vi "DataTranslation.vi"() -> ()   [LabVIEW 2014]
doc: "This vi will take data with multiple DT boxes for an arbitrary number of channels either differentially or single ended, depending upon how you have wired the boxes up."
uses:
  Controls/DT_Cluster.ctl
  Controls/DT_Mode.ctl
  Globals/Meas_global.vi
  Globals/Dynamic_call_global.ph.vi
  Globals/Trav_pos_global.vi
  Globals/Extra_Commands_Global.vi
  <userlib>/LV-Link3/PolySubVIs/DtCreateAinChan.vi
  <userlib>/LV-Link3/PolySubVIs/DtCreateCtrRateChan.vi
  <userlib>/LV-Link3/PolySubVIs/DtOLTimingSetInput.vi
  <userlib>/LV-Link3/PolySubVIs/DtOLStartNormal.vi
  <userlib>/LV-Link3/PolySubVIs/DtOLTriggerDigital.vi
  <userlib>/LV-Link3/PolySubVIs/DtOLReadMultiple2D.vi
panel:
  out "DAQ Error":errorcluster
  out "Array":T1[](array[typedef])
  out "Waveform Graph":dbl[][](graph)
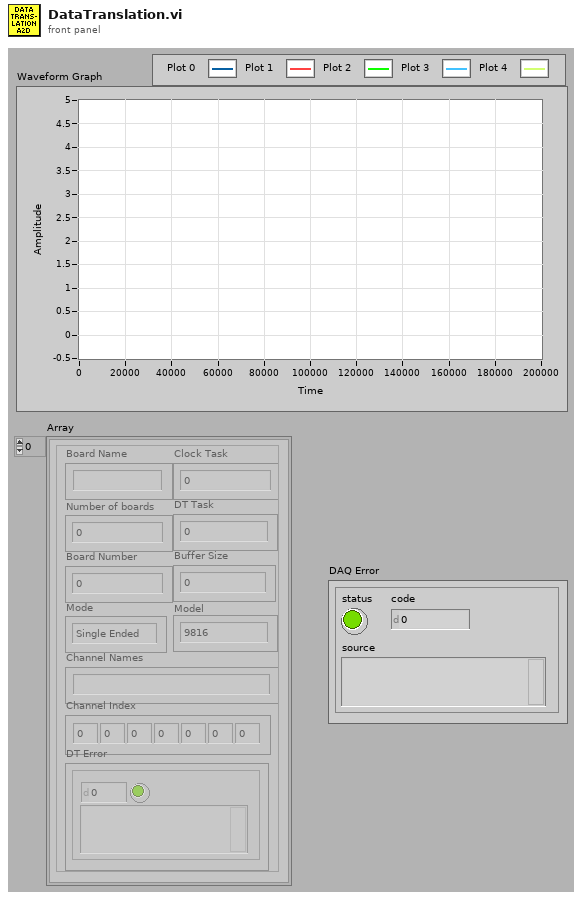
[diagram p1: front panel]
types:
  T1 = typedef "DT_Cluster.ctl" = cluster{"Board Name":string, "Number of boards":u32, "Board Number":u32, "Channel Names":string, "Channel Index":i32[], "DT Task":i32, "DT Error":errorcluster, "Mode":T2, "Buffer Size":u32, "Clock Task":i32, "Model":enum16{"9816", "9836", "9853"}}
  T2 = typedef "DT_Mode.ctl" = enum16{"Single Ended", "Differential"}
  T3 = typedef "Trigger_Mode.ctl" = enum16{"Free Running", "Start on Trigger", "Trigger Every Block", "Trigger Every Sample"}
  T4 = typedef "LDA_Setup.ctl" = cluster{"dimensions":enum16{"1D", "2D"}, "Analogue Freq Multiplier":dbl}
  T5 = enum32{"Internal Clock", "External Clock", "No Timing"}
  T6 = typedef "Traverse_cluster.ctl" = cluster{"Start X":dbl, "Start Y":dbl, "Start Z":dbl, "End X":dbl, "End Y":dbl, "End Z":dbl, "No. of pts.":i32, "Spacing":T7, "Filename":path, "Tunnel Speed":dbl, "Averaging time (min)":dbl, "Extra Commands":string, "Specific Arguments":string, "Emission Rate (l/min)":dbl, "Trace Gas Concentration (%)":dbl, "Density Ratio":string, "Comments":string, "Row No":i32, "Row Type Selector":T8, "Completion time":string, "Row Duration (mins)":dbl, "No. of Valid pts.":i32, "Meas Setup File":string}
  T7 = typedef "Spacing.ctl" = enum16{"Linear", "Log", "Gauss", "Specified", "N/A"}
  T8 = typedef "Multi_run_mode.ctl" = enum16{"Move Traverse Only", "Set Tunnel Speed Only", "Set Source Only", "Set Measurement Conditions", "Single Measurement", "Vertical Profile", "Lateral Profile", "Longitudinal Profile", "Explore Volume", "Multi-Axis Profile", "Auto Calibrate", "Meas Fast FID Bkgnd", "Check Beam Power", "Scanning Valve Measurement", "Run VI Named:", "Set ADAM Ch", "Wait (minutes)", "Send Message", "Synchronize With:", "Fall Back to this Row", "Turn Off Row Repeating", "Blank Row", "Traverse 3D Volume"}
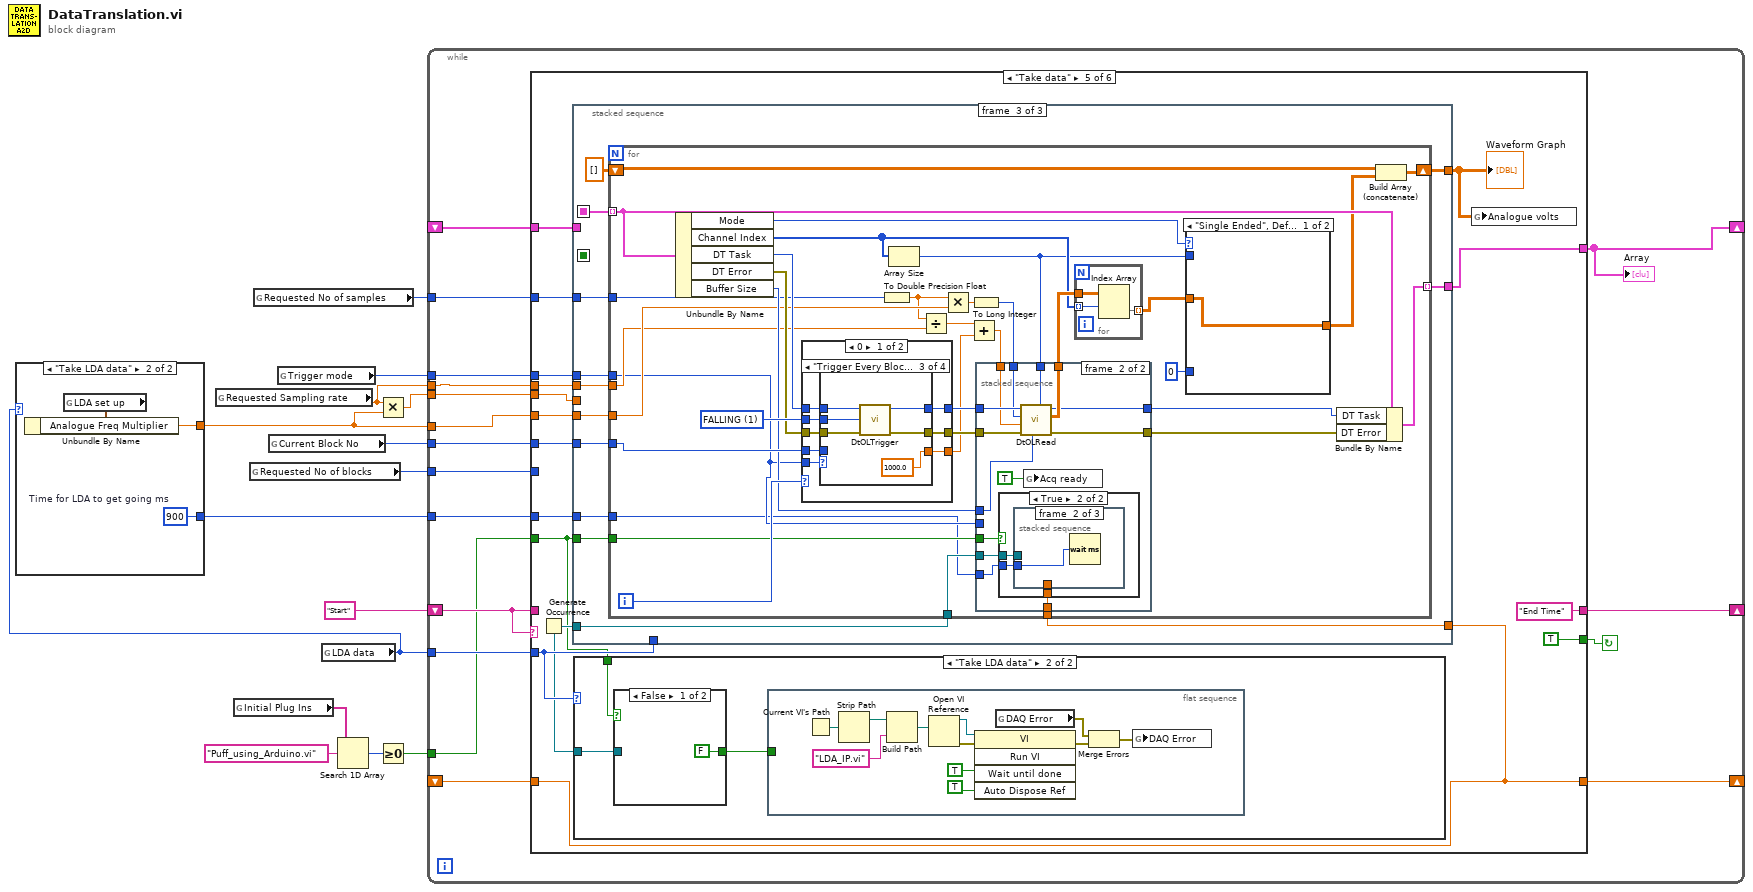
[diagram p0: block diagram]
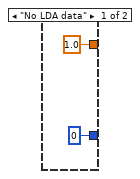
[diagram p2: hidden frame]
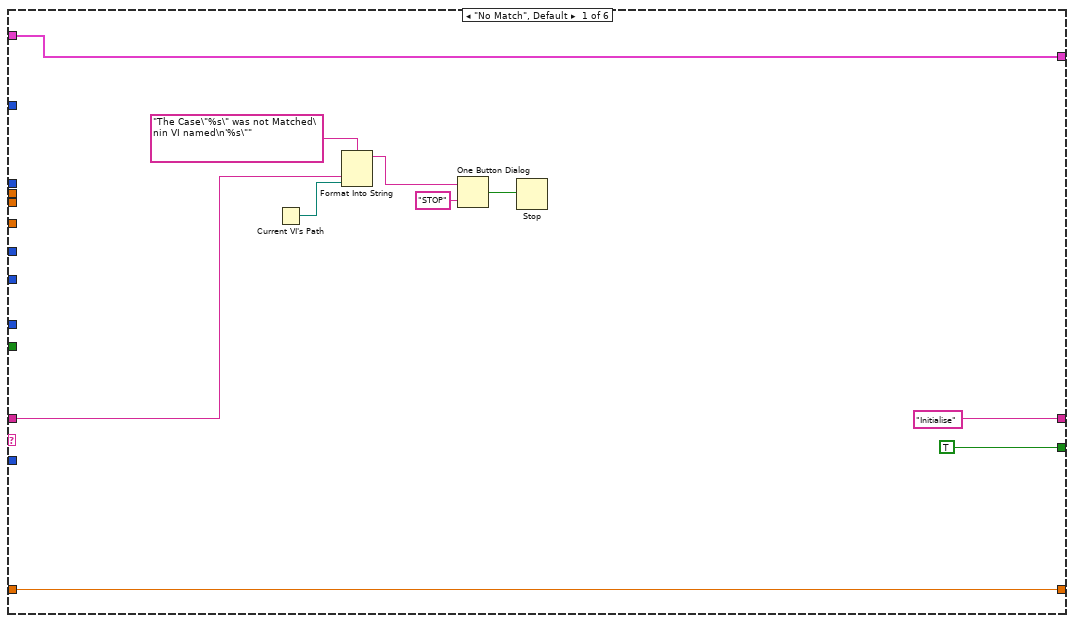
[diagram p3: hidden frame]
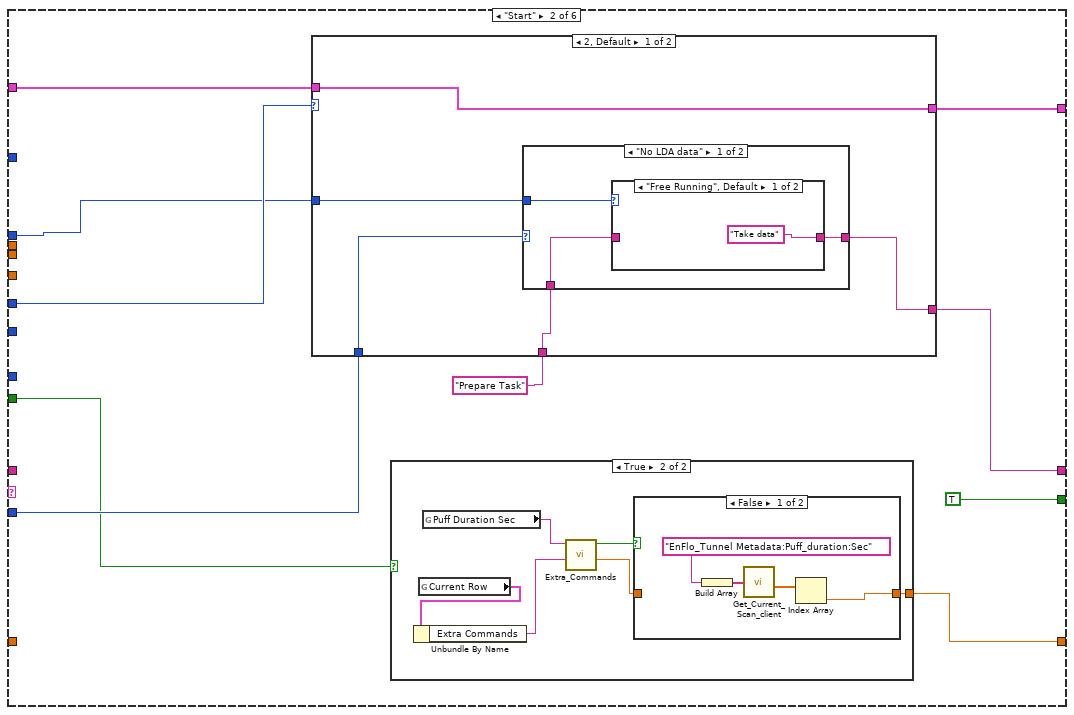
[diagram p4: hidden frame]
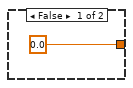
[diagram p5: hidden frame]
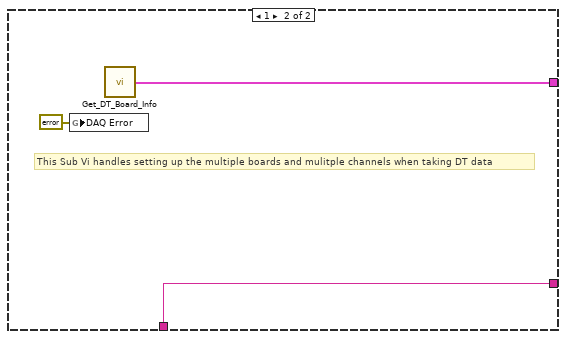
[diagram p9: hidden frame]
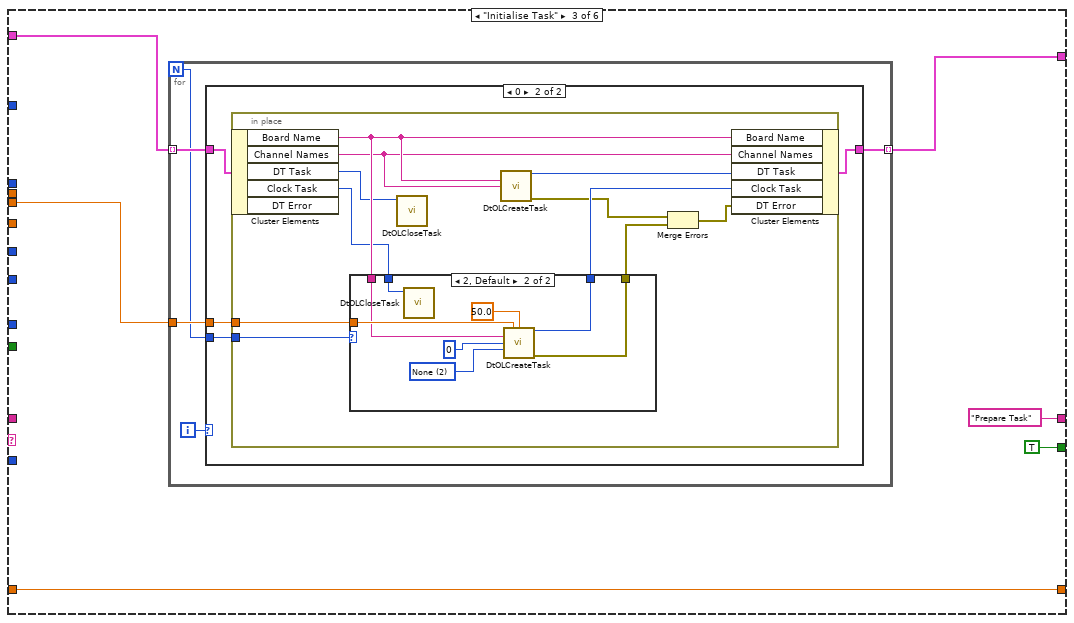
[diagram p10: hidden frame]
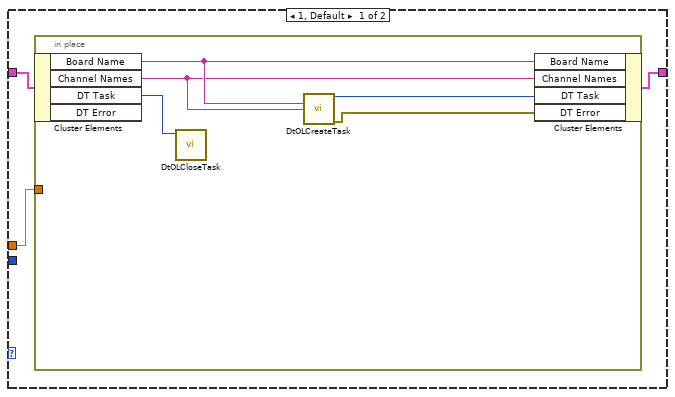
[diagram p11: hidden frame]
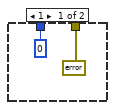
[diagram p12: hidden frame]
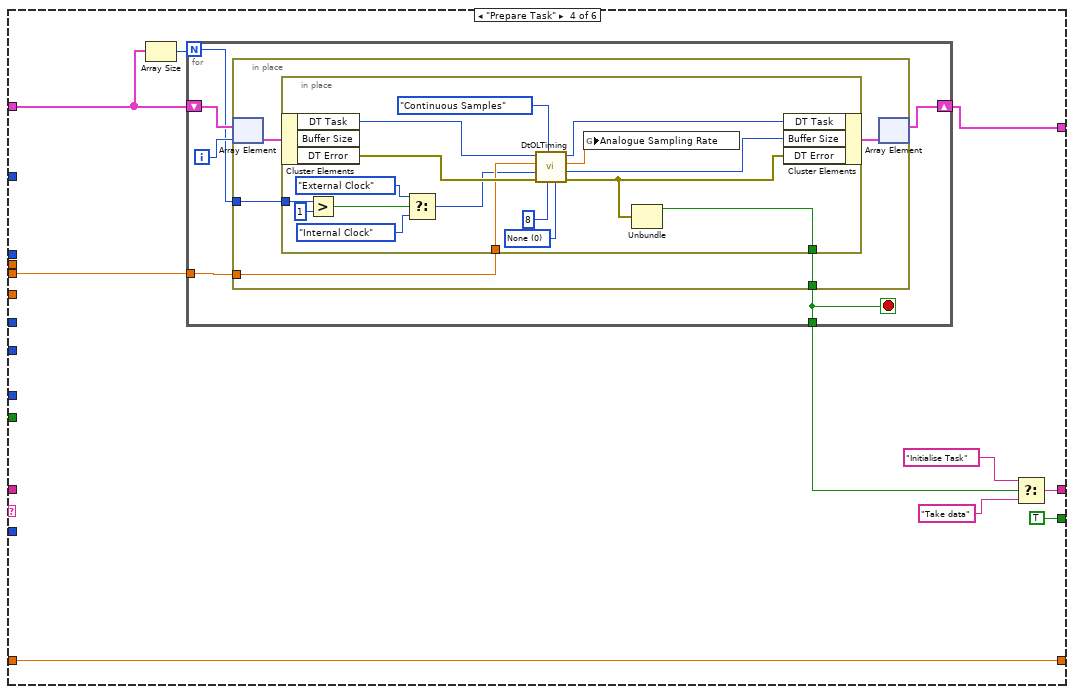
[diagram p13: hidden frame]
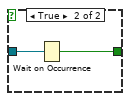
[diagram p15: hidden frame]
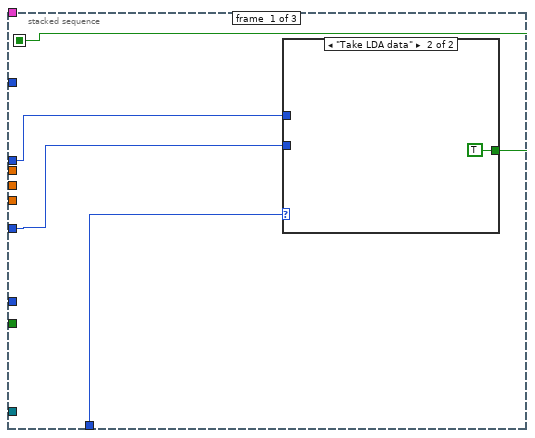
[diagram p16: hidden frame]
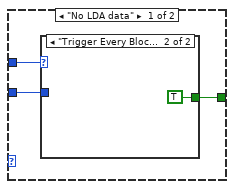
[diagram p17: hidden frame]
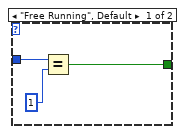
[diagram p18: hidden frame]
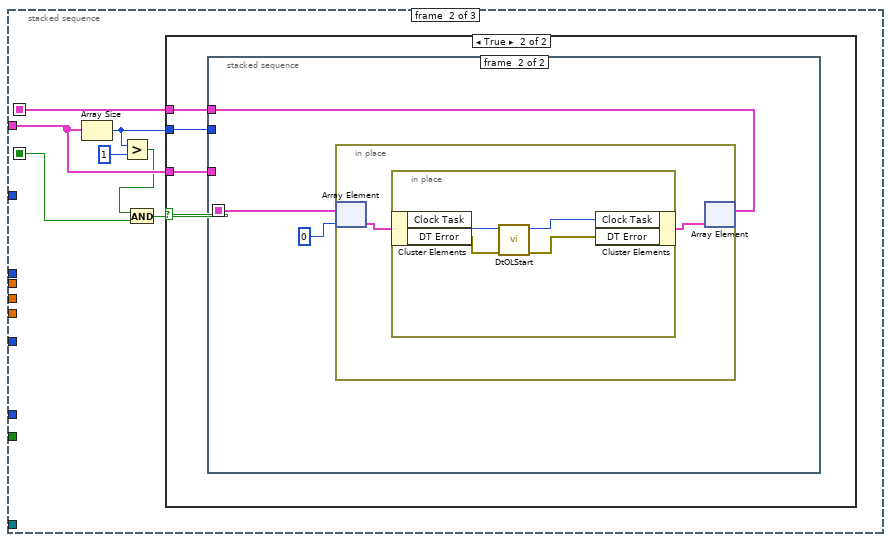
[diagram p19: hidden frame]
diagram:
  n1 = global read "Meas_global.vi" "Requested Sampling rate"() -> (w9:dbl)
  n2 = global read "Dynamic_call_global.ph.vi" "Initial Plug Ins"() -> (w5:string[])
  n3 = global read "Meas_global.vi" "Requested No of blocks"() -> (w8:i32)
  n4 = global read "Meas_global.vi" "Requested No of samples"() -> (w13:i32)
  n5 = global read "Meas_global.vi" "Current Block No"() -> (w11:i32)
  n6 = global read "Meas_global.vi" "Trigger mode"() -> (w12:T3)
  n7 = global read "Meas_global.vi" "LDA data"() -> (w6:enum16{"No LDA data", "Take LDA data"})
  n8 = case shown="\"Take LDA data\"" w6 {
    tunnel: [1.0 ("Analogue Freq Multiplier") w18] -> w7
    tunnel: [u32 0 ("Time for LDA to get going ms") w17] -> w1
    frame "No LDA data" {
    }
    frame "Take LDA data" {
      w17 = u32 900  # Time for LDA to get going ms
      n9 = global read "Meas_global.vi" "LDA set up"() -> (w19:T4)
      n10 = Unbundle By Name(w19) -> ("Analogue Freq Multiplier"=w18:dbl)
    }
  }
  n11 = Search 1D Array(1D array=w5, element="Puff_using_Arduino.vi") -> (index of element=w3:i32)  [unwired: 1 in]
  n12 = Multiply(x=w9, y=w7) -> (x*y=w10:dbl)
  n13 = Greater Or Equal To 0?(x=w3) -> (x >= 0?=w2:bool)
  n14 = while {
    shift-left: "Start" -> [w35]
    shift-right: [w36] -> _
    tunnel: w10 -> [w34]
    tunnel: w13 -> [w33]
    tunnel: w11 -> [w32]
    tunnel: w12 -> [w30]
    shift-right: [w29] -> _
    shift-left: _ -> [w28]
    tunnel: w6 -> [w27]
    tunnel: w7 -> [w26]
    tunnel: w9 -> [w25]
    tunnel: w8 -> [w24]
    tunnel: w2 -> [w23]
    shift-right: [w22] -> _
    shift-left: _ -> [w21]
    tunnel: w1 -> [w20]
    stop <- w31 continue-if-true
    n15 = case shown="\"Take data\"" w35 {
      tunnel: ["Initialise" w52 "Prepare Task" w133 "End Time" "" ("f")] -> w36
      tunnel: w35 -> [w42 _ _ _ _ _]
      tunnel: w34 -> [_ _ w86 w129 w170 _]
      tunnel: w33 -> [_ _ _ _ w179 _]
      tunnel: w32 -> [_ w53 _ _ w177 w371]
      tunnel: [TRUE TRUE TRUE TRUE TRUE FALSE] -> w31
      tunnel: w30 -> [_ w49 _ _ w176 _]
      tunnel: w28 -> [w38 w54 w84 w128 w175 w375]
      tunnel: [w38 w55 w85 w130 w174 w374] -> w29
      tunnel: w27 -> [_ w50 _ _ w169 _]
      tunnel: w26 -> [_ _ _ _ w172 _]
      tunnel: w25 -> [_ _ _ _ w171 _]
      tunnel: w24 -> [_ _ _ _ _ w372]
      tunnel: w23 -> [_ w48 _ _ w166 _]
      tunnel: [w37 w47 w83 w127 w167 w367] -> w22
      tunnel: w21 -> [w37 _ w83 w127 w167 w367]
      tunnel: w20 -> [_ _ _ _ w165 _]
      frame "No Match", Default {
        n16 = Current VI's Path() -> (path=w41:path)
        n17 = Format Into String(format string="The Case\"%s\" was not Matched\nin VI named\n'%s\"" ("Format String"), w42, w41) -> (resulting string=w45:string)  [unwired: 2 in, 1 out]
        n18 = One Button Dialog(message=w45, button name ("OK")="STOP") -> (true=w43:bool)
        n19 = Stop(stop? (T)=w43) -> ()
      }
      frame "Start" {
        n20 = case shown="2, Default" w53 {
          tunnel: [w73 w82] -> w55
          tunnel: w54 -> [w73 _]
          tunnel: [w71 w80] -> w52
          tunnel: "Prepare Task" -> [w70 w80]
          tunnel: w50 -> [w72 _]
          tunnel: w49 -> [w69 _]
          frame 2, Default {
            n21 = case shown="\"No LDA data\"" w72 {
              tunnel: [w76 w79] -> w71
              tunnel: w70 -> [w74 w79]
              tunnel: w69 -> [w75 _]
              frame "No LDA data" {
                n22 = case shown="\"Free Running\", Default" w75 {
                  tunnel: ["Take data" w78] -> w76
                  tunnel: w74 -> [_ w78]
                  frame "Free Running", Default {
                  }
                  frame "Trigger Every Block" {
                  }
                }
              }
              frame "Take LDA data" {
              }
            }
          }
          frame 1 {
            # "This Sub Vi handles setting up the multiple boards and mulitple channels when taking DT data"
            n23 = global write "Meas_global.vi" "DAQ Error"(errorcluster {"status"=FALSE, "code"=0, "source"=""} ("DAQ Error")) -> ()
            n24 = call "Get_DT_Board_Info.vi"() -> ("DT Cluster Array"=w82:T1[])  [unwired: 5 in]
          }
        }
        n25 = case shown="True" w48 {
          tunnel: [0.0 w63] -> w47
          frame False {
          }
          frame True {
            n26 = global read "Trav_pos_global.vi" "Current Row"() -> (w62:T6)
            n27 = Unbundle By Name(w62) -> ("Extra Commands"=w61:string)
            n28 = global read "Extra_Commands_Global.vi" "Puff Duration Sec"() -> (w60:string)
            n29 = call "Extra_Commands.vi"("String to Search"=w61, "Command"=w60) -> ("Numeric Value"=w58:dbl, "Command Found"=w59:bool)  [unwired: 2 in, 2 out]
            n30 = case shown="False" w59 {
              tunnel: [w64 w68] -> w63
              tunnel: w58 -> [_ w68]
              frame False {
                n31 = Build Array("EnFlo_Tunnel Metadata:Puff_duration:Sec") -> (w66:string[])
                n32 = call "Get_Current_Scan_client.vi"("ADAM Ch Names"=w66) -> ("Numerical Values"=w67:dbl[])  [unwired: 1 in, 2 out]
                n33 = Index Array(array=w67) -> (element=w64:dbl)  [unwired: 1 in]
              }
              frame True {
              }
            }
          }
        }
      }
      frame "Initialise Task" {
        n34 = for {
          N -> [w89]
          tunnel: w84 -> [w93] mode=indexing
          tunnel: w86 -> [w92]
          tunnel: [w91] -> w85 mode=indexing
          i -> [w90]
          n35 = case shown="0" w90 {
            tunnel: w93 -> [w96 w105]
            tunnel: w92 -> [w95 w104]
            tunnel: [w94 w103] -> w91
            tunnel: w89 -> [_ w102]
            frame 1, Default {
              n36 = in-place {
                in-place-border: w95 -> [_]
                n37 = in-place-cluster #1(w96) -> ("Board Name"=w101:string, "Channel Names"=w98:string, "DT Task"=w97:i32)  [unwired: 1 out]
                n38 = call <userlib>:"DtOLCloseTask.vi"("Task in"=w97) -> ()  [unwired: 10 in, 1 out]
                n39 = call-poly <userlib>:"DtOLCreateTask.vi"("Board Name"=w101, "Channel"=w98) -> ("Task out"=w100:i32, "error out"=w99:errorcluster)  [unwired: 11 in, 1 out]
                n40 = in-place-cluster #1("Board Name"=w101, "Channel Names"=w98, "DT Task"=w100, "DT Error"=w99) -> (w94:T1)
              }
            }
            frame 0 {
              n41 = in-place {
                in-place-border: w104 -> [w116]
                in-place-border: w102 -> [w107]
                n42 = in-place-cluster #2(w105) -> ("Board Name"=w114:string, "Channel Names"=w109:string, "DT Task"=w108:i32, "Clock Task"=w106:i32)  [unwired: 1 out]
                n43 = case shown="2, Default" w107 {
                  tunnel: w116 -> [_ w123]
                  tunnel: [errorcluster {"status"=FALSE, "code"=0, "source"=""} ("error out") w122] -> w115
                  tunnel: w114 -> [_ w121]
                  tunnel: [0 ("Task out") w120] -> w112
                  tunnel: w106 -> [_ w119]
                  frame 1 {
                  }
                  frame 2, Default {
                    w126 = 2 items=["LowLevel", "HighLevel", "None"] ("Gate Type")
                    n44 = call <userlib>:"DtOLCloseTask.vi"("Task in"=w119) -> ()  [unwired: 10 in, 1 out]
                    n45 = call-poly <userlib>:"DtOLCreateTask.vi"("Requested\nFrequency (Hz)"=w123, "Duty Cycle"=50.0, "Board Name"=w121, "Counter Num"=u32 0, "Gate Type"=w126) -> ("Task out"=w120:i32, "error out"=w122:errorcluster)  [unwired: 8 in, 1 out]
                  }
                }
                n46 = call <userlib>:"DtOLCloseTask.vi"("Task in"=w108) -> ()  [unwired: 10 in, 1 out]
                n47 = call-poly <userlib>:"DtOLCreateTask.vi"("Board Name"=w114, "Channel"=w109) -> ("Task out"=w113:i32, "error out"=w111:errorcluster)  [unwired: 11 in, 1 out]
                n48 = Merge Errors(w111, w115) -> (w110:errorcluster)
                n49 = in-place-cluster #2("Board Name"=w114, "Channel Names"=w109, "DT Task"=w113, "Clock Task"=w112, "DT Error"=w110) -> (w103:T1)
              }
            }
          }
        }
      }
      frame "Prepare Task" {
        n50 = Array Size(array=w128) -> (size(s)=w132:i32)
        n51 = for {
          N: w132 -> [w137]
          shift-right: [w139] -> w130
          shift-left: w128 -> [w141]
          tunnel: [w142] -> w131
          tunnel: w129 -> [w138]
          i -> [w140]
          stop <- w142 stop-if-true
          n52 = in-place {
            in-place-border: [w147] -> w142
            in-place-border: w138 -> [w144]
            in-place-border: w137 -> [w143]
            n53 = in-place-array #3(w141, w140) -> (w146:T1)
            n54 = in-place {
              in-place-border: [w158] -> w147
              in-place-border: w144 -> [w157]
              in-place-border: w143 -> [w156]
              w149 = 0 items=["None", "Master", "Slave"] ("Sync Mode")
              n55 = in-place-cluster #4(w146) -> ("DT Task"=w163:i32, "DT Error"=w162:errorcluster)  [unwired: 1 out]
              n56 = Greater?(x=w156, y=1) -> (0:w154:bool)
              n57 = Select(t=T5."External Clock" ("Timing"), s=w154, f=T5."Internal Clock" ("Timing")) -> (s? t:f=w151:T5)
              n58 = call-poly <userlib>:"DtOLTiming.vi"("Sync Mode"=w149, "Num Buffers"=u32 8, "Sample Mode"=enum16{"Finite Samples", "Continuous Samples"}."Continuous Samples", "error in (no error)"=w162, "Timing"=w151, "Sample Freq (Hz)"=w157, "Task in"=w163) -> ("error out"=w159:errorcluster, "Buffer Size"=w161:u32, "Actual Sample Freq"=w164:dbl, "Task out"=w160:i32)  [unwired: 1 in]
              n59 = global write "Meas_global.vi" "Analogue Sampling Rate"(w164) -> ()
              n60 = Unbundle(w159) -> ("status"=w158:bool)  [unwired: 2 out]
              n61 = in-place-cluster #4("DT Task"=w160, "Buffer Size"=w161, "DT Error"=w159) -> (w145:T1)
            }
            n62 = in-place-array #3(w145) -> (w139:T1[])  [unwired: 1 out]
          }
        }
        n63 = Select(t="Initialise Task", s=w131, f="Take data") -> (s? t:f=w133:string)
      }
      frame "Take data" {
        n64 = Generate Occurrence() -> (w168:refnum<k4>)
        n65 = stacked-sequence {
          seq-local: [_ w216 _] -> [_ _ w246]
          seq-local: [w199 _ _] -> [_ w211 _]
          tunnel: w179 -> [_ _ w254]
          tunnel: w177 -> [w200 _ w253]
          tunnel: w176 -> [w198 _ w252]
          tunnel: w175 -> [_ w215 _]
          tunnel: [_ _ w251] -> w174
          tunnel: [_ _ w249] -> w173
          tunnel: w172 -> [_ _ w248]
          tunnel: w171 -> [_ _ w247]
          tunnel: w169 -> [w201 _ _]
          tunnel: w170 -> [_ _ _]
          tunnel: w168 -> [_ _ w245]
          tunnel: w166 -> [_ _ w244]
          tunnel: w167 -> [_ _ w243]
          tunnel: w165 -> [_ _ w242]
          frame #0 {
            n66 = case shown="\"Take LDA data\"" w201 {
              tunnel: w200 -> [w204 _]
              tunnel: [w203 TRUE] -> w199
              tunnel: w198 -> [w202 _]
              frame "No LDA data" {
                n67 = case shown="\"Trigger Every Block\"" w202 {
                  tunnel: w204 -> [w207 _]
                  tunnel: [w205 TRUE] -> w203
                  frame "Free Running", Default {
                    n68 = Equal?(x=w207, y=1) -> (x = y?=w205:bool)
                  }
                  frame "Trigger Every Block" {
                  }
                }
              }
              frame "Take LDA data" {
              }
            }
          }
          frame #1 {
            n69 = Array Size(array=w215) -> (size(s)=w214:i32)
            n70 = Greater?(x=w214, y=1) -> (0:w212:bool)
            n71 = And(x=w212, y=w211) -> (x .and. y?=w210:bool)
            n72 = case shown="True" w210 {
              tunnel: [w217 w220] -> w216
              tunnel: w215 -> [w217 w219]
              tunnel: w214 -> [_ w218]
              frame False {
              }
              frame True {
                n73 = stacked-sequence {
                  seq-local: [w221 _] -> [_ w234]
                  tunnel: [_ w233] -> w220
                  tunnel: w219 -> [w223 _]
                  tunnel: w218 -> [w222 _]
                  frame #0 {
                    n74 = for {
                      N: w222 -> [_]
                      shift-right: [w224] -> w221
                      shift-left: w223 -> [w225]
                      i -> [w226]
                      n75 = in-place {
                        n76 = in-place-array #5(w225, w226) -> (w228:T1)
                        n77 = in-place {
                          n78 = in-place-cluster #6(w228) -> ("DT Task"=w232:i32, "DT Error"=w231:errorcluster)
                          n79 = call-poly <userlib>:"DtOLStart.vi"("error in (no error)"=w231, "Task in"=w232) -> ("error out"=w230:errorcluster, "Task out"=w229:i32)  [unwired: 8 in]
                          n80 = in-place-cluster #6("DT Task"=w229, "DT Error"=w230) -> (w227:T1)
                        }
                        n81 = in-place-array #5(w227) -> (w224:T1[])  [unwired: 1 out]
                      }
                    }
                  }
                  frame #1 {
                    n82 = in-place {
                      n83 = in-place-array #7(w234, 0) -> (w237:T1)
                      n84 = in-place {
                        n85 = in-place-cluster #8(w237) -> ("Clock Task"=w240:i32, "DT Error"=w241:errorcluster)
                        n86 = call-poly <userlib>:"DtOLStart.vi"("error in (no error)"=w241, "Task in"=w240) -> ("error out"=w238:errorcluster, "Task out"=w239:i32)  [unwired: 8 in]
                        n87 = in-place-cluster #8("Clock Task"=w239, "DT Error"=w238) -> (w236:T1)
                      }
                      n88 = in-place-array #7(w236) -> (w233:T1[])  [unwired: 1 out]
                    }
                  }
                }
              }
            }
          }
          frame #2 {
            n89 = for {
              tunnel: w254 -> [w269]
              tunnel: w253 -> [w287]
              tunnel: w252 -> [w256]
              tunnel: w246 -> [w283] mode=indexing
              tunnel: [w282] -> w251 mode=indexing
              shift-right: [w279] -> w249
              shift-left: dbl[][] [] -> [w278]
              tunnel: w248 -> [w268]
              tunnel: w247 -> [w266]
              tunnel: w245 -> [w259]
              tunnel: w244 -> [w258]
              tunnel: w243 -> [w257]
              tunnel: w242 -> [w255]
              i -> [w276]
              w288 = 1 items=["RISING", "FALLING"] ("External Trigger Polarity")
              n90 = Unbundle By Name(w283) -> ("Mode"=w273:T2, "Channel Index"=w280:i32[], "DT Task"=w286:i32, "DT Error"=w285:errorcluster, "Buffer Size"=w271:u32)
              n91 = case shown="0" w276 {
                tunnel: [w332 w363] -> w289
                tunnel: w288 -> [w331 _]
                tunnel: w287 -> [w330 _]
                tunnel: w256 -> [w329 _]
                tunnel: w286 -> [w328 w363]
                tunnel: w285 -> [w327 w362]
                tunnel: [w326 w362] -> w284
                tunnel: [w325 10.0 ("x")] -> w263
                frame 0 {
                  n92 = case shown="\"Trigger Every Block\"" w329 {
                    tunnel: [w335 w340 w355 w360] -> w332
                    tunnel: w328 -> [w335 w341 w357 w360]
                    tunnel: w330 -> [_ w342 _ _]
                    tunnel: w331 -> [_ w339 w356 _]
                    tunnel: w327 -> [w334 w338 w354 w359]
                    tunnel: [w334 w337 w353 w359] -> w326
                    tunnel: [10.0 ("x") w336 1000.0 ("x") 1000.0 ("x")] -> w325
                    frame "Free Running" {
                    }
                    frame "Start on Trigger" {
                      n93 = case shown="1" w342 {
                        tunnel: w341 -> [w348 w351]
                        tunnel: w338 -> [w347 w350]
                        tunnel: [w345 w351] -> w340
                        tunnel: [w346 w350] -> w337
                        tunnel: w339 -> [w344 _]
                        tunnel: [1000.0 ("x") 10.0 ("x")] -> w336
                        frame 1 {
                          n94 = call-poly <userlib>:"DtOLTrigger.vi"("error in (no error)"=w347, "External Trigger Polarity"=w344, "Task in"=w348) -> ("error out"=w346:errorcluster, "Task out"=w345:i32)  [unwired: 7 in]
                        }
                        frame 2, Default {
                        }
                      }
                    }
                    frame "Trigger Every Block" {
                      n95 = call-poly <userlib>:"DtOLTrigger.vi"("error in (no error)"=w354, "External Trigger Polarity"=w356, "Task in"=w357) -> ("error out"=w353:errorcluster, "Task out"=w355:i32)  [unwired: 7 in]
                    }
                    frame "Trigger Every Sample" {
                    }
                  }
                }
                frame 1, Default {
                }
              }
              n96 = To Double Precision Float(number=w269) -> (double precision float=w261:dbl)
              n97 = Array Size(array=w280) -> (size(s)=w262:i32)
              n98 = Divide(x=w261, y=w266) -> (x/y=w264:dbl)
              n99 = Multiply(x=w261, y=w268) -> (x*y=w267:dbl)
              n100 = Add(x=w264, y=w263) -> (x+y=w277:dbl)
              n101 = To Long Integer(number=w267) -> (32bit integer=w260:i32)
              n102 = stacked-sequence {
                tunnel: w289 -> [_ w306]
                tunnel: w284 -> [_ w305]
                tunnel: [_ w304] -> w281
                tunnel: w277 -> [_ w303]
                tunnel: [_ w302] -> w275
                tunnel: w271 -> [_ w298]
                tunnel: [_ w301] -> w270
                tunnel: w260 -> [_ w300]
                tunnel: w262 -> [_ w299]
                tunnel: w259 -> [_ w296]
                tunnel: w258 -> [_ w295]
                tunnel: w257 -> [_ w294]
                tunnel: w256 -> [w291 _]
                tunnel: w255 -> [w290 w293]
                frame #0 {
                  n103 = case shown="\"Free Running\"" w291 {
                    tunnel: w290 -> [w292 _]
                    frame "Free Running" {
                      n104 = Wait (ms)(milliseconds to wait=w292) -> ()  [unwired: 1 out]
                    }
                    frame Default {
                    }
                  }
                }
                frame #1 {
                  n105 = case shown="True" w295 {
                    tunnel: w296 -> [_ w309]
                    tunnel: w294 -> [_ w308]
                    tunnel: w293 -> [_ w307]
                    frame False {
                    }
                    frame True {
                      n106 = stacked-sequence {
                        tunnel: w309 -> [w310 _ _]
                        tunnel: w308 -> [_ _ w312]
                        tunnel: w307 -> [_ w311 _]
                        frame #0 {
                          n107 = Set Occurrence(w310) -> ()
                        }
                        frame #1 {
                          n108 = Wait (ms)(milliseconds to wait=w311) -> ()  [unwired: 1 out]
                        }
                        frame #2 {
                          n109 = call "Puff_using_Arduino_oneshot.vi"("Puff_duration:Sec"=w312) -> ()  [unwired: 7 in]
                        }
                      }
                    }
                  }
                  n110 = call-poly <userlib>:"DtOLRead.vi"("Number Chan to Read"=w299, "Buffer size"=w298, "error in (no error)"=w305, "Timeout"=w303, "Samples Per Channel"=w300, "Task in"=w306) -> ("error out"=w301:errorcluster, "2D Data out"=w304:dbl[][], "Task out"=w302:i32)  [unwired: 1 in, 2 out]
                  n111 = global write "Meas_global.vi" "Acq ready"(TRUE ("Acq ready")) -> ()
                }
              }
              n112 = for {
                tunnel: w280 -> [w366] mode=indexing
                tunnel: w281 -> [w365]
                tunnel: [w364] -> w265 mode=indexing
                n113 = Index Array(array=w365, index (row)=w366) -> (element=w364:dbl[])  [unwired: 1 in]
              }
              n114 = case shown="\"Single Ended\", Default" w273 {
                tunnel: w265 -> [w313 w318]
                tunnel: [w313 w317] -> w274
                tunnel: 0 ("size(s)") -> [_ w316]
                tunnel: w262 -> [_ w315]
                frame "Single Ended", Default {
                }
                frame "Differential" {
                  n115 = expression code="0.5*x"(w315) -> (w314:i32)
                  n116 = for {
                    N: w314 -> [_]
                    tunnel: w318 -> [w324]
                    shift-right: [w323] -> _
                    shift-left: w316 -> [w322]
                    tunnel: [w320] -> w317 mode=indexing
                    n117 = Index Array(array=w324, index (row) #1=w322) -> (element #1=w319:dbl[], element #2=w321:dbl[])  [unwired: 3 in]
                    n118 = expression code="x+2"(w322) -> (w323:i32)
                    n119 = Subtract(x=w319, y=w321) -> (x-y=w320:dbl[])
                  }
                }
              }
              n120 = Bundle By Name(cluster=w283, "DT Task"=w275, "DT Error"=w270) -> (w282:T1)
              n121 = Build Array (concatenate)(w278, w274) -> (w279:dbl[][])
            }
          }
        }
        "Waveform Graph" <- w173
        n122 = case shown="\"Take LDA data\"" w169 {
          tunnel: w168 -> [_ w183]
          tunnel: w166 -> [_ w181]
          frame "No LDA data", Default {
          }
          frame "Take LDA data" {
            n123 = case shown="False" w181 {
              tunnel: w183 -> [_ w186]
              tunnel: [FALSE ("timed out") w185] -> w182
              frame False {
              }
              frame True {
                n124 = Wait on Occurrence(2:w186) -> (0:w185:bool)  [unwired: 2 in]
              }
            }
            n125 = flat-sequence {
              tunnel: w182 -> [_]
              frame #0 {
                n126 = Current VI's Path() -> (path=w191:path)
                n127 = Strip Path(path=w191) -> (stripped path=w187:path)  [unwired: 1 out]
                n128 = Build Path(base path=w187, name or relative path="LDA_IP.vi") -> (appended path=w192:path)
                n129 = Open VI Reference(vi path=w192) -> (vi reference=w195:refnum<vi>, error out=w196:errorcluster)  [unwired: 5 in]
                n130 = invoke class="VI" method="Run VI"(reference=w195, error in=w196, "Wait until done"=TRUE ("Wait Until Done"), "Auto Dispose Ref"=TRUE ("Wait until done")) -> (error out=w189:errorcluster)  [unwired: 1 in, 4 out]
                n131 = global read "Meas_global.vi" "DAQ Error"() -> (w190:errorcluster)
                n132 = Merge Errors(w190, w189) -> (w188:errorcluster)
                n133 = global write "Meas_global.vi" "DAQ Error"(w188) -> ()
              }
            }
          }
        }
        n134 = global write "Meas_global.vi" "Analogue volts"(w173) -> ()
      }
      frame "End Time" {
        n135 = Equal?(x=w371, y=w372) -> (x = y?=w369:bool)
        n136 = case shown="True" w369 {
          tunnel: w375 -> [w378 w380]
          tunnel: [w378 w379] -> w374
          frame False {
          }
          frame True {
            n137 = for {
              N -> [w381]
              tunnel: w380 -> [w384] mode=indexing
              tunnel: [w383] -> w379 mode=indexing
              i -> [w382]
              n138 = case shown="0" w382 {
                tunnel: w384 -> [w386 w393]
                tunnel: [w385 w392] -> w383
                tunnel: w381 -> [_ w391]
                frame 1, Default {
                  n139 = in-place {
                    n140 = in-place-cluster #9(w386) -> ("DT Task"=w390:i32, "DT Error"=w389:errorcluster)
                    n141 = call <userlib>:"DtOLCloseTask.vi"("Error in"=w389, "Task in"=w390) -> ("Error Out"=w388:errorcluster)  [unwired: 9 in]
                    n142 = in-place-cluster #9("DT Task"=0, "DT Error"=w388) -> (w385:T1)
                  }
                }
                frame 0 {
                  n143 = in-place {
                    in-place-border: w391 -> [w394]
                    n144 = in-place-cluster #10(w393) -> ("DT Task"=w400:i32, "DT Error"=w399:errorcluster, "Clock Task"=w397:i32)
                    n145 = case shown="2, Default" w394 {
                      tunnel: [errorcluster {"status"=FALSE, "code"=0, "source"=""} ("Error Out") w405] -> w402
                      tunnel: w397 -> [_ w404]
                      frame 1 {
                      }
                      frame 2, Default {
                        n146 = call <userlib>:"DtOLCloseTask.vi"("Task in"=w404) -> ("Error Out"=w405:errorcluster)  [unwired: 10 in]
                      }
                    }
                    n147 = call <userlib>:"DtOLCloseTask.vi"("Error in"=w399, "Task in"=w400) -> ("Error Out"=w398:errorcluster)  [unwired: 9 in]
                    n148 = Merge Errors(w398, w402) -> (w401:errorcluster)
                    n149 = in-place-cluster #10("DT Task"=0, "DT Error"=w401, "Clock Task"=0) -> (w392:T1)
                  }
                }
              }
            }
          }
        }
        n150 = global write "Meas_global.vi" "Acq ready"(FALSE ("Acq ready")) -> ()
        n151 = global read "Meas_global.vi" "DAQ Error"() -> (w370:errorcluster)
        n152 = for {
          tunnel: w374 -> [w409] mode=indexing
          shift-right: [w406] -> w373
          shift-left: w370 -> [w407]
          n153 = Unbundle By Name(w409) -> ("DT Error"=w408:errorcluster)
          n154 = Merge Errors(w407, w408) -> (w406:errorcluster)
        }
        "DAQ Error" <- w373
        n155 = global write "Meas_global.vi" "DAQ Error"(w373) -> ()
      }
    }
    "Array" <- w29
  }
